vi "parseAttributeData.vi"(8 "error in (no error)":errorcluster, 10 "XMLString in":string, 11 "AttributeReader In":refnum<class "XMLAttributeParser.lvclass">) -> (0 "error out":errorcluster, 2 "attributeData":T1(array[cluster]), 3 "AttributeReader Out":refnum<class "XMLAttributeParser.lvclass">)   [LabVIEW 2014, in "XML.lvlib" / "XMLAttributeParser.lvclass"]
doc: "This is the main Parse Attrbute method that calls the separate parsing of type and value methods and then combines the results."
uses:
  <userlib>/Common/XML/XMLAttributeParser/XMLAttributeParser.lvclass
  <userlib>/Common/XML/Typedefs/AttributeElements.ctl
  <userlib>/Common/XML/XMLAttributeParser/removeEmptyArrayElement.vi
  <userlib>/Common/XML/XMLAttributeParser/removeQuotations.vi
  <userlib>/Common/XML/XMLAttributeParser/replaceSingleQuotes.vi
  <userlib>/Common/XML/XML.lvlib
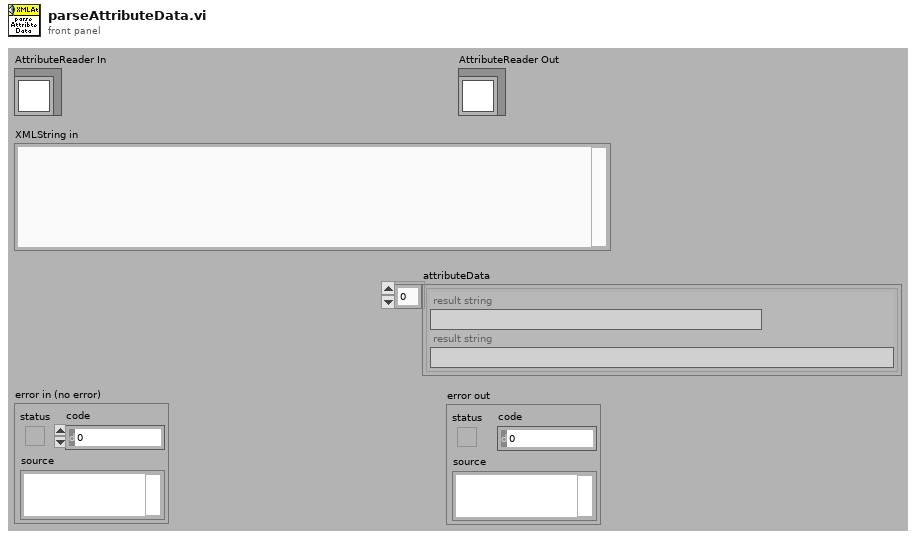
[diagram p1: front panel]
types:
  T1 = cluster{"result string":string, "result string":string}[]
  T2 = typedef "XML.lvlib/AttributeElements.ctl" = cluster{"attributeType":string, "attributeValue":string}
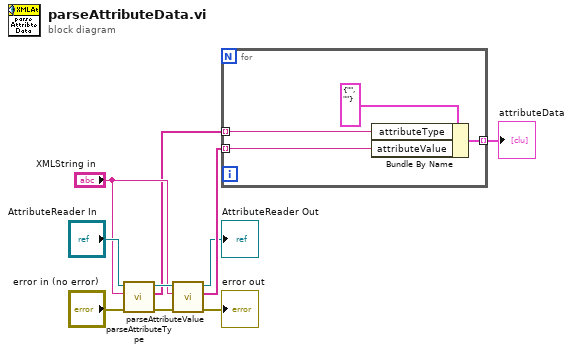
[diagram p0: block diagram]
diagram:
  n1 = call <userlib>:"parseAttributeType.vi"("error in (no error)"="error in (no error)", "XML in"="XMLString in", "AttributeReader in"="AttributeReader In") -> ("error out"=w6:errorcluster, "ParsedTypes"=w3:string[], "AttributeReader out"=w9:refnum<class "XMLAttributeParser.lvclass">)  [unwired: 6 in]
  n2 = call <userlib>:"parseAttributeValue.vi"("error in (no error)"=w6, "XMLString in"="XMLString in", "AttributeReader in"=w9) -> ("error out"=→"error out":errorcluster, "ParsedValues"=w4:string[], "AttributeReader out"=→"AttributeReader Out":refnum<class "XMLAttributeParser.lvclass">)  [unwired: 6 in]
  n3 = for {
    tunnel: [w13] -> w2 mode=indexing
    tunnel: w4 -> [w12] mode=indexing
    tunnel: w3 -> [w11] mode=indexing
    n4 = Bundle By Name(cluster=T2 {"attributeType"="", "attributeValue"=""} ("attributeData"), "attributeType"=w11, "attributeValue"=w12) -> (w13:T2)
  }
  "attributeData" <- w2
